vi "Control-UserScript.vi"(8 "Error In":errorcluster, 11 "DCM-DSI.lvclass":refnum<class "DCM-DSI.lvclass">) -> (0 "Error Out":errorcluster, 3 "DCM-DSI.lvclass":refnum<class "DCM-DSI.lvclass">)   [LabVIEW 2016, in "DSI-RT.lvlib"]
uses:
  DSI-RT.lvlib
  Classes/DCM-DSI/DCM-DSI.lvclass
  Shared/Typedefs/Engine-Channel.ctl
  Classes/DCM-DSI/Read Channels.vi
  Classes/DCM-DSI/Write Channels.vi
  <vilib>/addons/Software Calibration Management/xSCM/CalPoint.xnode
  <vilib>/gmath/NI_Gmath.lvlib
  <vilib>/addons/Software Calibration Management/xSCM/ni_scm.dll
  Shared/DSI-Shared.lvlib
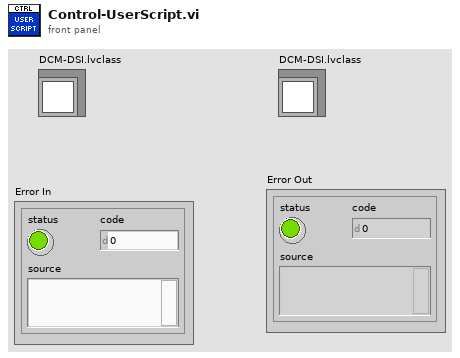
[diagram p1: front panel]
types:
  T1 = typedef "DSI-Shared.lvlib/Engine-Channel.ctl" = cluster{"Name":string, "Unit":string, "Value":sgl}
  T2 = cluster{"Y Values":dbl[][], "Tables":i32[][][], "Variables input decode":i32[], "Variables output decode":i32[]}
  T3 = cluster{"Name":string, "Unit":string, "Value":sgl}[]
  T4 = typedef "DCM-DSI.lvclass/Channel.ctl" = cluster{"Name":string, "Unit":string, "Value":sgl}
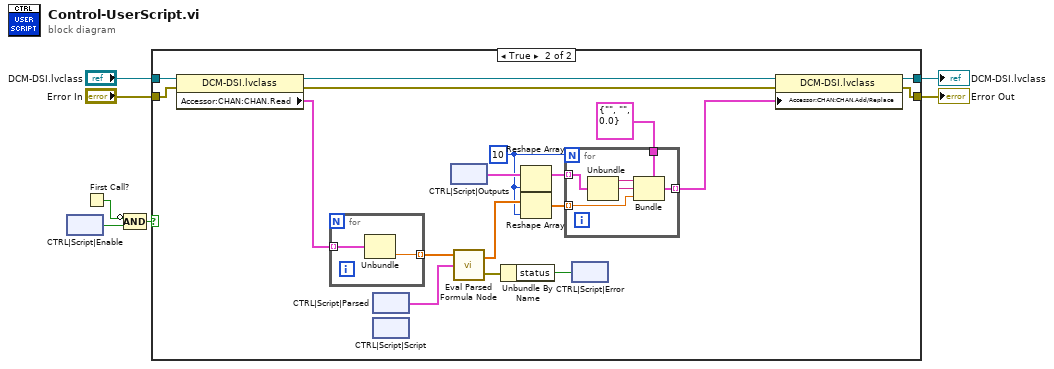
[diagram p0: block diagram]
diagram:
  n1 = xnode "CTRL|Script|Enable"() -> ("Value"=w1:bool)
  n2 = First Call?() -> (First Call?: T/F=w2:bool)
  n3 = Compound Arithmetic op=AND(invert w2, w1) -> (w3:bool)
  n4 = case shown="True" w3 {
    tunnel: "DCM-DSI.lvclass" -> [w9 w27]
    tunnel: [w9 w24] -> w6
    tunnel: [w8 w23] -> w5
    tunnel: "Error In" -> [w8 w22]
    frame False {
    }
    frame True {
      w13 = 10
      n5 = property class="DCM-DSI.lvclass"(reference=w27, error in=w22) -> (reference out=w26:refnum<class "DCM-DSI.lvclass">, error out=w25:errorcluster, "Accessor:CHAN:CHAN.Read"=w21:T4[])
      n6 = for {
        tunnel: w21 -> [w58] mode=indexing
        tunnel: [w57] -> w11 mode=indexing
        n7 = Unbundle(w58) -> ("Value"=w57:sgl)  [unwired: 2 out]
      }
      n8 = xnode "CTRL|Script|Parsed"() -> ("Value"=w20:T2)
      n9 = xnode "CTRL|Script|Script"() -> ()  [unwired: 1 out]
      n10 = xnode "CTRL|Script|Outputs"() -> ("Value"=w16:T3)
      n11 = call <vilib>:"Eval Parsed Formula Node.vi"("Parsed Formula Node"=w20, "Input Values"=w11) -> ("error out"=w19:errorcluster, "Output Values"=w17:dbl[])  [unwired: 1 in]
      n12 = Unbundle By Name(w19) -> ("status"=w18:bool)
      n13 = Reshape Array(w16, w13) -> (w15:T3)
      n14 = Reshape Array(w17, w13) -> (w14:dbl[])
      n15 = for {
        N: w13 -> [_]
        tunnel: w14 -> [w84] mode=indexing
        tunnel: w15 -> [w82] mode=indexing
        tunnel: [w83] -> w10 mode=indexing
        tunnel: T1 {"Name"="", "Unit"="", "Value"=0.0} ("Channel In") -> [w79]
        n16 = Unbundle(w82) -> ("Name"=w81:string, "Unit"=w80:string)  [unwired: 1 out]
        n17 = Bundle(cluster=w79, "Name"=w81, "Unit"=w80, "Value"=w84) -> (w83:T1)
      }
      n18 = xnode "CTRL|Script|Error"("Value"=w18) -> ()
      n19 = property class="DCM-DSI.lvclass"(reference=w26, error in=w25, "Accessor:CHAN:CHAN.Add/Replace"=w10) -> (reference out=w24:refnum<class "DCM-DSI.lvclass">, error out=w23:errorcluster)
    }
  }
  "DCM-DSI.lvclass" <- w6
  "Error Out" <- w5
